vi "FTW-CodeGen-RegenerateAfterAdapt.vi"(5 "Previous Adapted Types":variant[](array[variant]), 7 "Adaptive Terminals (that Trigger Regen on Datatype Change)":string[](array[string]), 9 "Wired Terminals":cluster{"Type":variant, "ID":string}[](array[cluster])) -> (6 "Current Adapted Types":variant[](array[variant]), 8 "Reply":string[](array[string]))   [LabVIEW 2015]
uses:
  FTW-CodeGen-XNodeReplyType.ctl
panel:
  # "Inputs"
  # "Outputs"
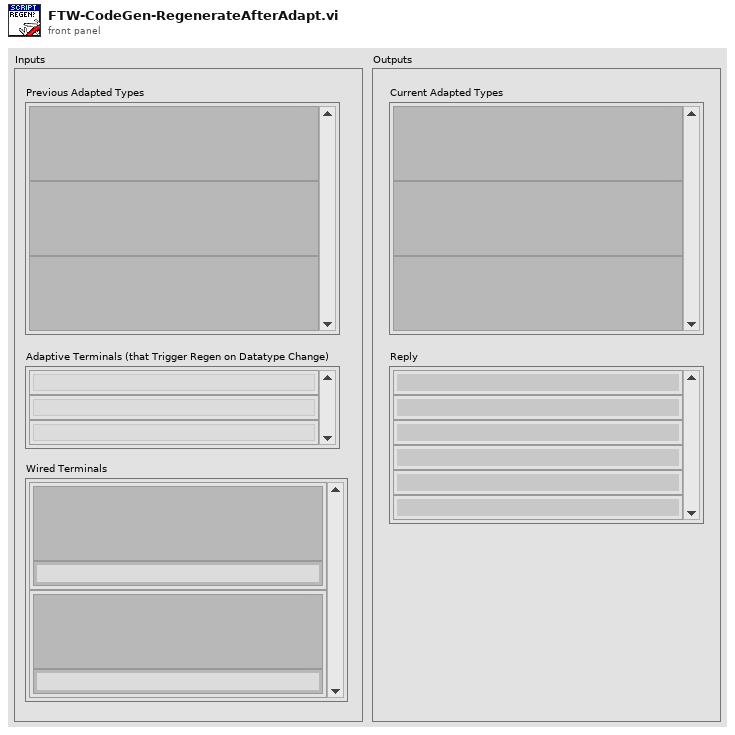
[diagram p1: front panel]
types:
  T1 = typedef "FTW-CodeGen-XNodeReplyType.ctl" = enum16{"UpdateState", "AdaptToInputs", "AdaptAndAugment", "CosmeticUpdate", "NoReply"}
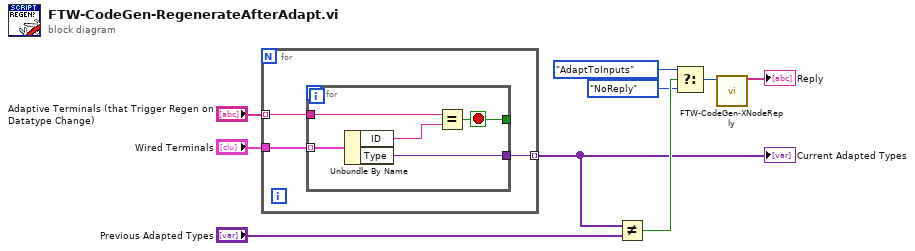
[diagram p0: block diagram]
diagram:
  n1 = for {
    tunnel: "Wired Terminals" -> [w12]
    tunnel: "Adaptive Terminals (that Trigger Regen on Datatype Change)" -> [w11] mode=indexing
    tunnel: [w10] -> w1 mode=indexing
    n2 = for {
      tunnel: [w17] -> w10
      tunnel: [w16] -> _
      tunnel: w12 -> [w15] mode=indexing
      tunnel: w11 -> [w13]
      stop <- w16 stop-if-true
      n3 = Unbundle By Name(w15) -> ("ID"=w14:string, "Type"=w17:variant)
      n4 = Equal?(x=w13, y=w14) -> (x = y?=w16:bool)
    }
  }
  "Current Adapted Types" <- w1
  n5 = Not Equal?(x=w1, y="Previous Adapted Types") -> (x != y?=w6:bool)
  n6 = Select(t=FTW-CodeGen-XNodeReplyType."AdaptToInputs" ("XNode Reply Type"), s=w6, f=FTW-CodeGen-XNodeReplyType."NoReply" ("XNode Reply Type")) -> (s? t:f=w3:T1)
  n7 = call "FTW-CodeGen-XNodeReply.vi"("XNode Reply Type"=w3) -> ("Reply"=→"Reply":string[])  [unwired: 14 in]
